vi "CIF Generate Top Level.vi"() -> ()   [LabVIEW 2021, in "Plugin Generator.lvlib"]
uses:
  Plugin Generator.lvlib
  <vilib>/CIF Foundation/CIF LabVIEW Scripting/LV Scripting/Typedef/Icon Overlay.ctl
  <vilib>/CIF Foundation/CIF Core/Channels/ChannelRegistrar/typedef/Channel Definition for Scripting.ctl
  <vilib>/CIF Foundation/CIF Channels Core/CIFChannels/Typedef/Direction.ctl
  <vilib>/CIF Foundation/CIF Core/Channels/ChannelRegistrar/typedef/Registered Channel Types.ctl
  Typedef/Documentation Info.ctl
  <vilib>/CIF Foundation/CIF LabVIEW Scripting/LV Scripting/LV Scripting Utilities.lvlib
  <vilib>/CIF Foundation/CIF Channels Core/CIFChannels/CIFChannels.lvclass
  <vilib>/CIF Foundation/CIF Core/Channels/ChannelRegistrar/ChannelRegistrar.lvlib
panel:
  in  "Documentation":T1
  in  "Channels to Create":T2[](array[typedef])
  in  "Icon Overlay":T5={"Text"="cifrock", "Background color"=7208704, "Text color"=0}
  out "error out":errorcluster
  in  "New Name":string="CIFRocks"
  in  "Copied Template Project Path":path=path "C:/Users/Public/Documents/LabVIEW Data/CIF/CIFRocks/Tests/Template Interactive Test.lvproj"
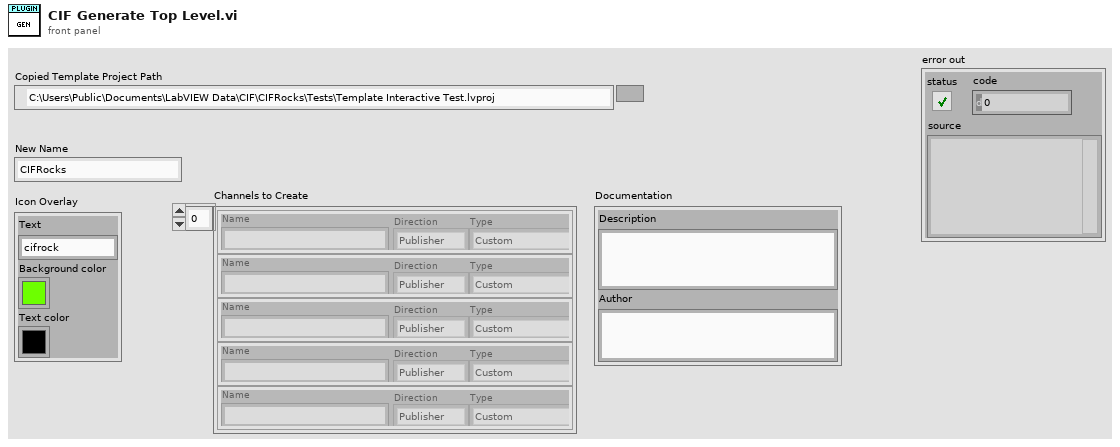
[diagram p1: front panel]
types:
  T1 = typedef "Plugin Generator.lvlib/Documentation Info.ctl" = cluster{"Description":string, "Author":string}
  T2 = typedef "ChannelRegistrar.lvlib/Channel Definition for Scripting.ctl" = cluster{"Name":string, "Direction":T3, "Type":T4}
  T3 = typedef "CIFChannels.lvclass/Direction.ctl" = enum16{"Publisher", "Subscriber"}
  T4 = typedef "ChannelRegistrar.lvlib/Registered Channel Types.ctl" = enum16{"Custom", "Double_Tag", "I64_Tag", "U64_Tag", "U8_FIFO", "CAN_FIFO", "L2Enet_FIFO", "DAQ_FIFO", "Universal_FIFO", "String_Tag"}
  T5 = typedef "LV Scripting Utilities.lvlib/Icon Overlay.ctl" = cluster{"Text":string, "Background color":u32, "Text color":u32}
  T6 = typedef "Plugin Generator.lvlib/Proto Names.ctl" = cluster{"PascalCase":string, "snake_case":string}
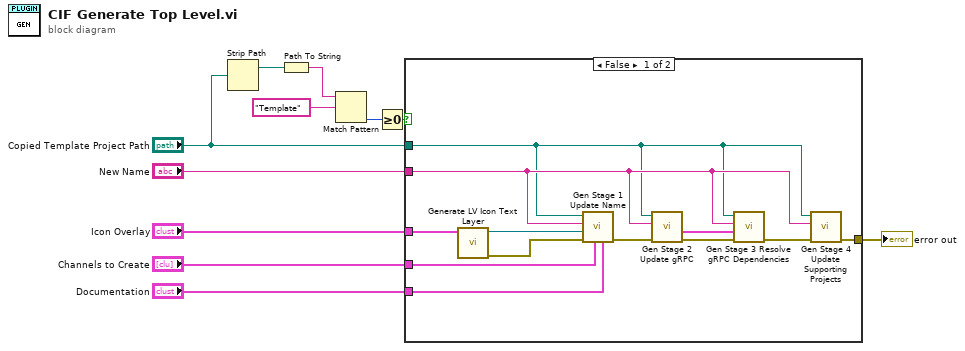
[diagram p0: block diagram]
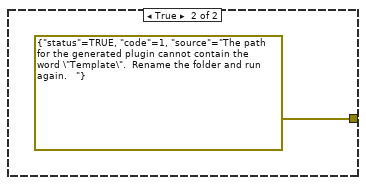
[diagram p2: hidden frame]
diagram:
  n1 = Strip Path(path="Copied Template Project Path") -> (stripped path=w8:path)  [unwired: 1 out]
  n2 = Path To String(path=w8) -> (string=w7:string)
  n3 = Match Pattern(string=w7, regular expression="Template") -> (offset past match=w5:i32)  [unwired: 1 in, 3 out]
  n4 = Greater Or Equal To 0?(x=w5) -> (x >= 0?=w4:bool)
  n5 = case shown="False" w4 {
    tunnel: [w21 errorcluster {"status"=TRUE, "code"=1, "source"="The path for the generated plugin cannot contain the word \"Template\".  Rename the folder and run again.   "} ("error out")] -> w11
    tunnel: "New Name" -> [w20 _]
    tunnel: "Copied Template Project Path" -> [w19 _]
    tunnel: "Icon Overlay" -> [w17 _]
    tunnel: "Channels to Create" -> [w18 _]
    tunnel: "Documentation" -> [w12 _]
    frame False {
      n6 = call <vilib>:"Generate LV Icon Text Layer.vi"("Icon Overlay"=w17) -> ("error out"=w15:errorcluster, "Icon.lvlclass out"=w16:refnum<class "Icon.lvclass">)  [unwired: 8 in, 1 out]
      n7 = call "Gen Stage 1 Update Name.vi"("Documentation"=w12, "Channels to Create"=w18, "error in"=w15, "Overlay Icon"=w16, "New Subname"=w20, "Template Project Path"=w19) -> ("error out"=w23:errorcluster)  [unwired: 5 in]
      n8 = call "Gen Stage 2 Update gRPC.vi"("error in"=w23, "New Subname"=w20, "Template Project Path"=w19) -> ("error out"=w22:errorcluster, "Proto Names"=w14:T6)  [unwired: 7 in]
      n9 = call "Gen Stage 3 Resolve gRPC Dependencies.vi"("error in"=w22, "Proto Names"=w14, "New Subname"=w20, "Template Project Path"=w19) -> ("error out"=w13:errorcluster)  [unwired: 7 in]
      n10 = call "Gen Stage 4 Update Supporting Projects.vi"("error in (no error)"=w13, "New Name"=w20, "Template Project Path"=w19) -> ("error out"=w21:errorcluster)  [unwired: 8 in]
    }
    frame True {
    }
  }
  "error out" <- w11
